vi "verify_Commands.vi"(0 "Command":string, 1 "error in":errorcluster) -> (2 "Command Found":bool, 3 "Command out":string, 4 "error out":errorcluster)   [LabVIEW 2015]
uses:
  <vilib>/Utility/error.llb/DialogType.ctl
  <userlib>/_OpenG.lib/array/array.llb/Search 1D Array (String)__ogtk.vi
  <userlib>/_OpenG.lib/array/array.llb/Empty 1D Array (I32)__ogtk.vi
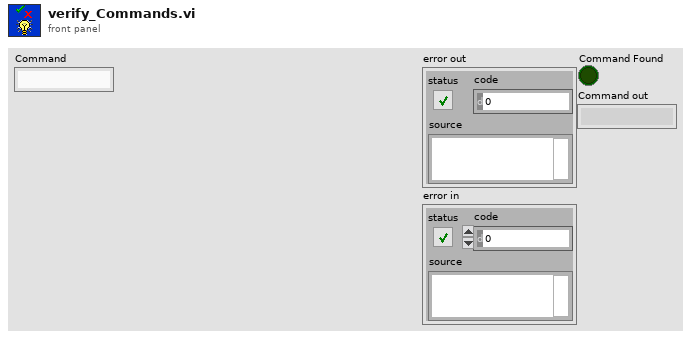
[diagram p1: front panel]
types:
  T1 = typedef "NI STM.lvlib/MetaDataElement.ctl" = string
  T2 = typedef "DialogType.ctl" = u16
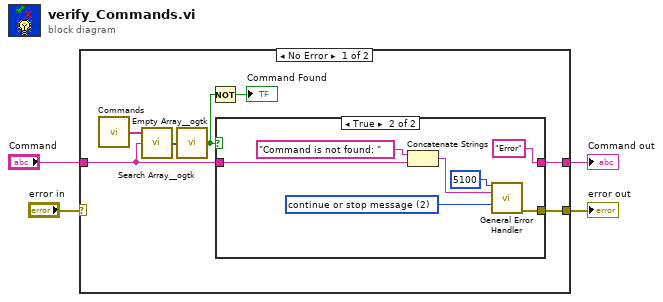
[diagram p0: block diagram]
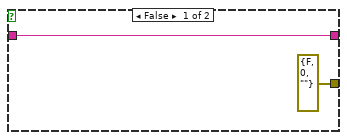
[diagram p2: hidden frame]
diagram:
  n1 = case shown="No Error" "error in" {
    selector: "error in" -> [_ w22]
    tunnel: [w9 w22] -> w4
    tunnel: "Command" -> [w6 w21]
    tunnel: [w5 w21] -> w1
    frame No Error {
      n2 = call "Commands.vi"() -> ("Commands"=w11:T1[])
      n3 = call-poly <userlib>:"Search Array__ogtk.vi"("Array"=w11, "Element Data"=w6) -> ("Indices of Elements"=w10:i32[])  [unwired: 7 in]
      n4 = call-poly <userlib>:"Empty Array__ogtk.vi"("Array"=w10) -> ("Empty Array?"=w8:bool)  [unwired: 8 in]
      n5 = Not(x=w8) -> (.not. x?=→"Command Found":bool)
      n6 = case shown="True" w8 {
        tunnel: w6 -> [w12 w17]
        tunnel: [errorcluster {"status"=FALSE, "code"=0, "source"=""} ("error out") w15] -> w9
        tunnel: [w12 "Error" ("source")] -> w5
        frame False {
        }
        frame True {
          w20 = T2 2 items=["no dialog", "OK message", "continue or stop message", "OK message + warnings", "continue/stop + warnings"] ("type of dialog (OK msg:1)")
          n7 = Concatenate Strings("Command is not found: " ("String to Prepend to source (\"\")"), w17) -> (w16:string)
          n8 = call <vilib>:"General Error Handler.vi"("[error code] (0)"=5100 ("code"), "[error source] (\" \")"=w16, "type of dialog (OK msg:1)"=w20) -> ("error out"=w15:errorcluster)  [unwired: 8 in, 4 out]
        }
      }
    }
    frame Error {
    }
  }
  "error out" <- w4
  "Command out" <- w1
